vi "HK Channel Setup and Test.vi"() -> ()   [LabVIEW 2019]
uses:
  HK Table/HK Current Value Table Settings.ctl
  HK Item/HK Channel Units and Setup.ctl
  HK Item/HK Channel enum Data Type.ctl
  HK Item/HK Channel Settings Physical.ctl
  HK Item/HK Channel Settings Scaling.ctl
  HK Item/HK Channel enum Scaling Type.ctl
  HK Item/HK Channel Settings Limits.ctl
  HK Alarms/HK Channel Settings Alarms.ctl
  HK Alarms/HK Alarm enum Action.ctl
  HK Table/HK Table.lvclass
  HK Item/HK Item.lvclass
  HK Table/HK Table.lvclass/HK Table.ctl
  HK Item/HK Item.lvclass/HK Item.ctl
  HK Alarms/HK Alarms.lvclass/HK Alarms.ctl
  HK Item/HK Channel Read Name.vi
  HK Table/HK Channel Write Channel Configuration File.vi
  HK Alarms/HK Alarms.lvclass
panel:
  in  "Channels":i32(listbox)
  in  "Tab Control":T1(tab)
  in  "Channel List":i32(listbox)
  in  "CVT Settings":T2 {"Max Age" format="%<%H:%M:%S>t"}
  in  "HK File":string
  in  "Save Button":bool
  in  "Update Ch":bool
  in  "Channel Name":string
  in  "Channel Setup":T3
  in  "Add Channel":bool
  in  "Update Phy":bool
  in  "Physical":T5
  in  "Scaling":T6
  in  "Update Alarms":bool
  in  "Limits":T8
  in  "Alarms":T9[](array[typedef])
  in  "Delete Channel":bool
  in  "Close":bool
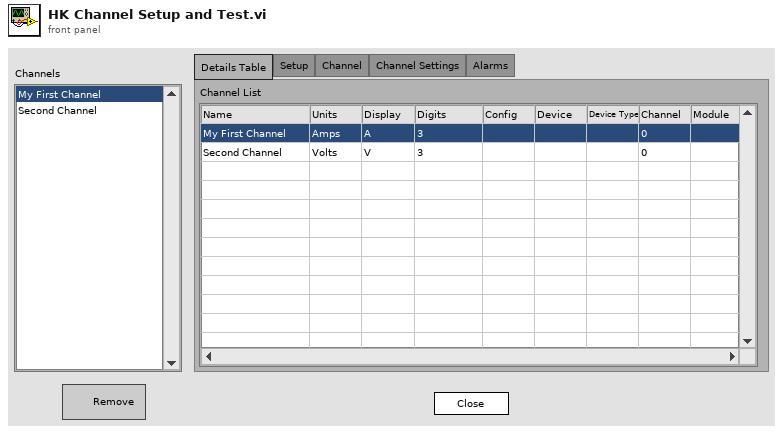
[diagram p1: front panel]
types:
  T1 = enum32{"Details Table", "Setup", "Channel", "Channel Settings", "Alarms"}
  T2 = typedef "HK Table.lvclass/HK Current Value Table Settings.ctl" = cluster{"Running Avg Elements":i32, "Max Age":dbl}
  T3 = typedef "HK Item.lvclass/HK Channel Units and Setup.ctl" = cluster{"Unit Type":string, "Units":string, "Configuration":string, "Digits":i32, "Data Type":T4}
  T4 = typedef "HK Item.lvclass/HK Channel enum Data Type.ctl" = enum16{"Floating Point", "Integer", "Enum", "String", "Waveform", "File"}
  T5 = typedef "HK Item.lvclass/HK Channel Settings Physical.ctl" = cluster{"Type":string, "Device":string, "Module":string, "Channel":i32}
  T6 = typedef "HK Item.lvclass/HK Channel Settings Scaling.ctl" = cluster{"Scaling Type":T7, "Parameters":dbl[]}
  T7 = typedef "HK Item.lvclass/HK Channel enum Scaling Type.ctl" = enum16{"None", "Polynomial"}
  T8 = typedef "HK Item.lvclass/HK Channel Settings Limits.ctl" = cluster{"Low Red":dbl, "Low Yellow":dbl, "Hi Yellow":dbl, "Hi Red":dbl}
  T9 = typedef "HK Item.lvclass/HK Channel Settings Alarms.ctl" = cluster{"Enabled":bool, "Deadband":i32, "Action":T10}
  T10 = typedef "HK Item.lvclass/HK Alarm enum Action.ctl" = enum16{"Light", "Message", "Safe"}
  T11 = cluster{"state":refnum<user-event>, "HK Channels":refnum<class "HK Table.lvclass">, "Channel Ref":refnum<class "HK Item.lvclass">}
  T12 = typedef "HK cluster Create Defaults.ctl" = cluster{"HK File":string, "CVT Settings":T2}
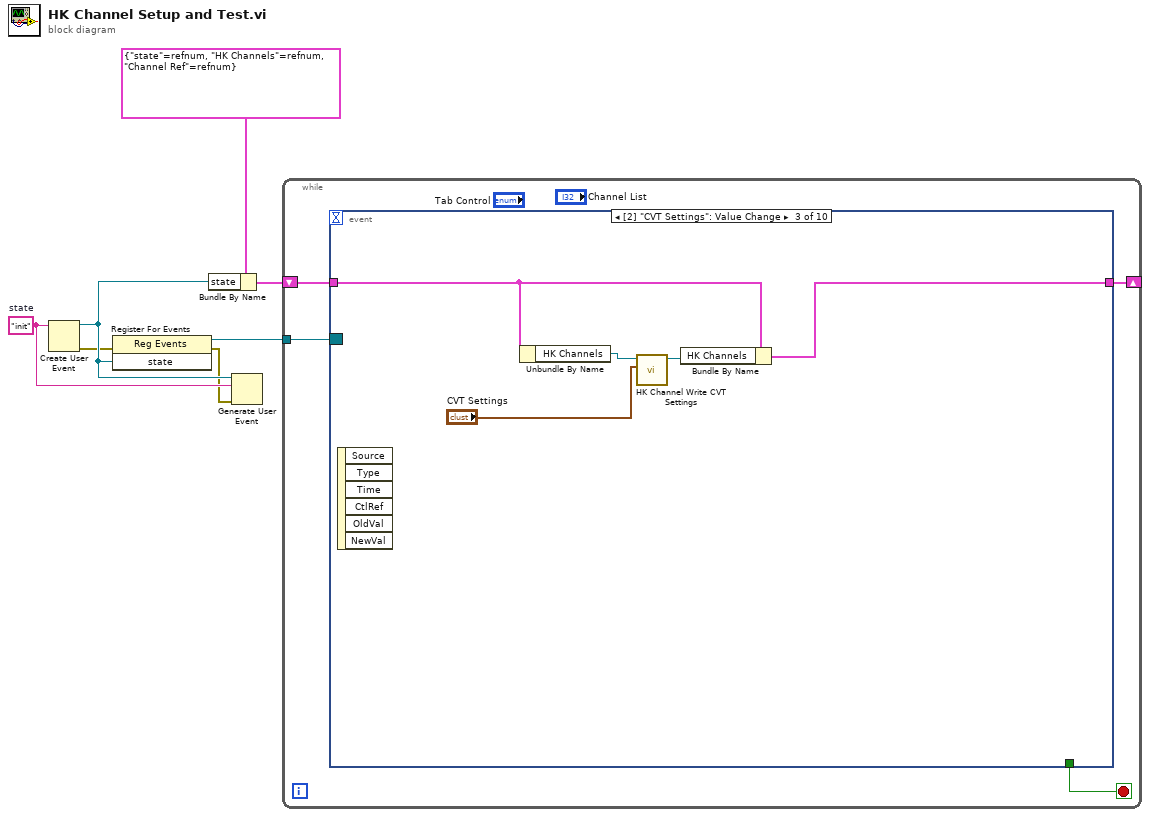
[diagram p0: block diagram]
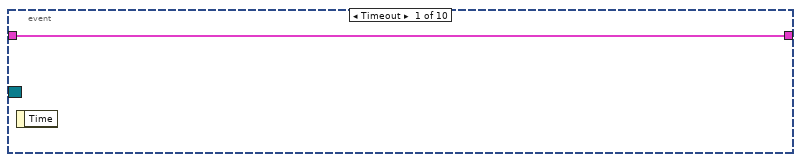
[diagram p2: hidden frame]
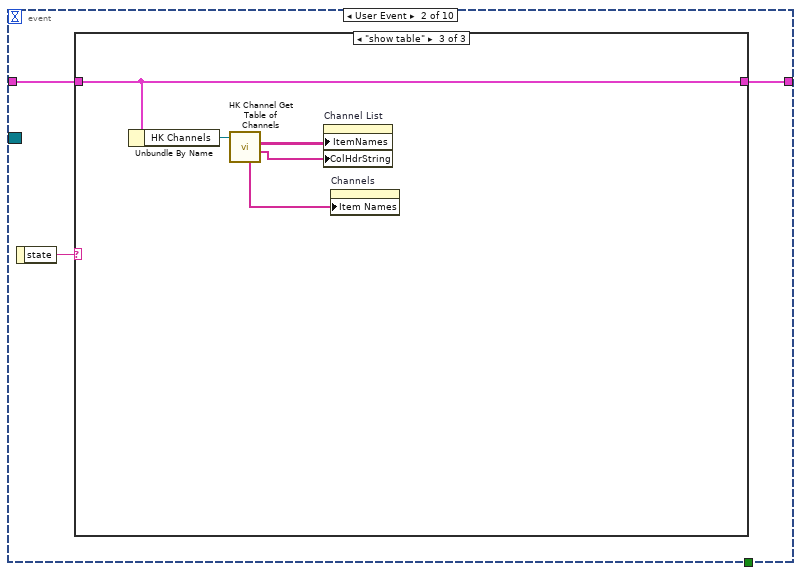
[diagram p3: hidden frame]
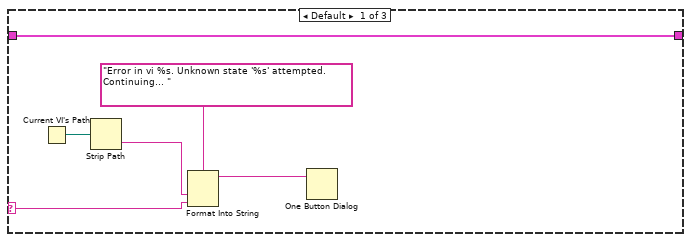
[diagram p4: hidden frame]
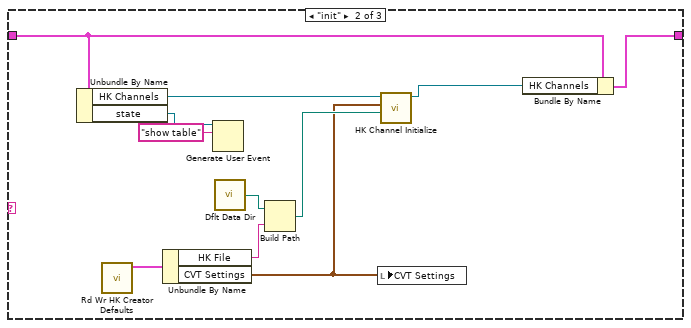
[diagram p5: hidden frame]
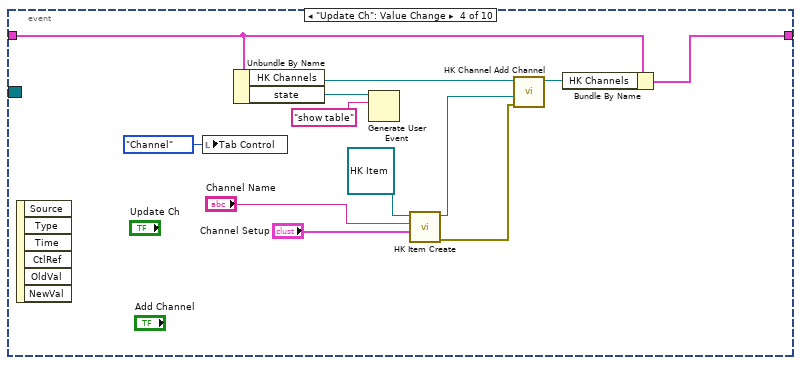
[diagram p6: hidden frame]
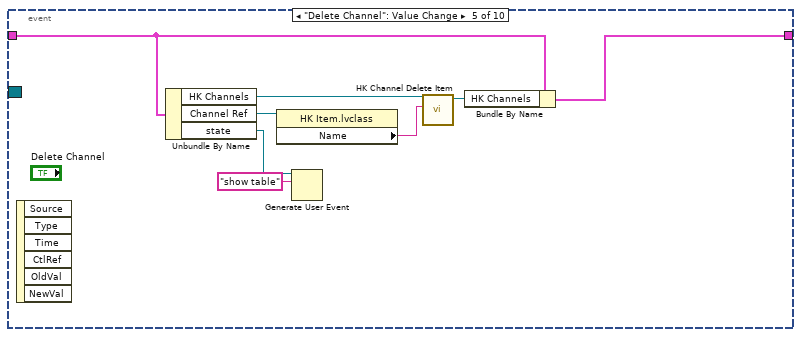
[diagram p7: hidden frame]
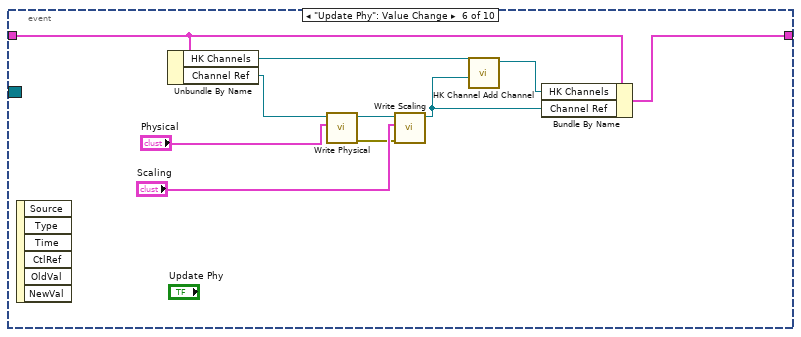
[diagram p8: hidden frame]
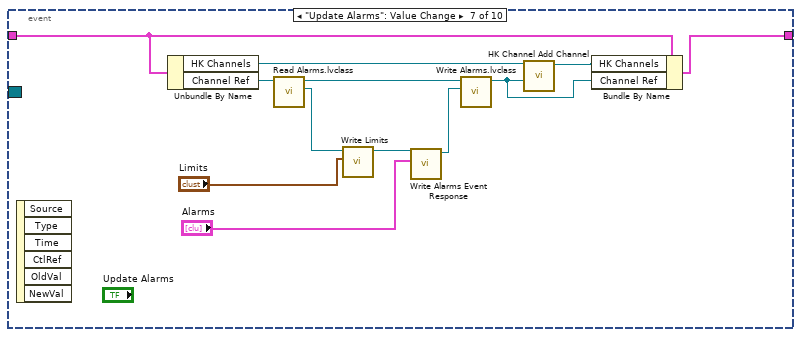
[diagram p9: hidden frame]
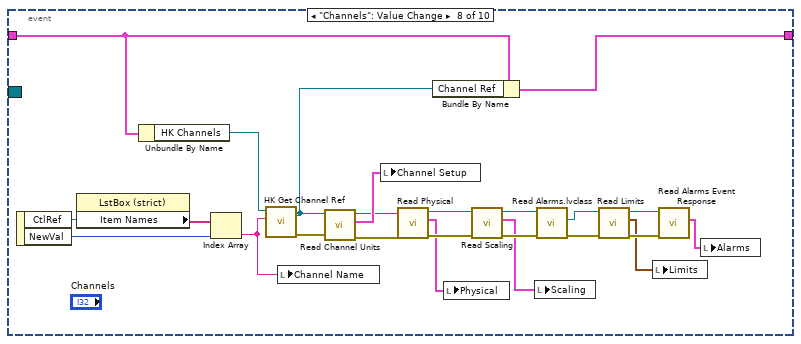
[diagram p10: hidden frame]
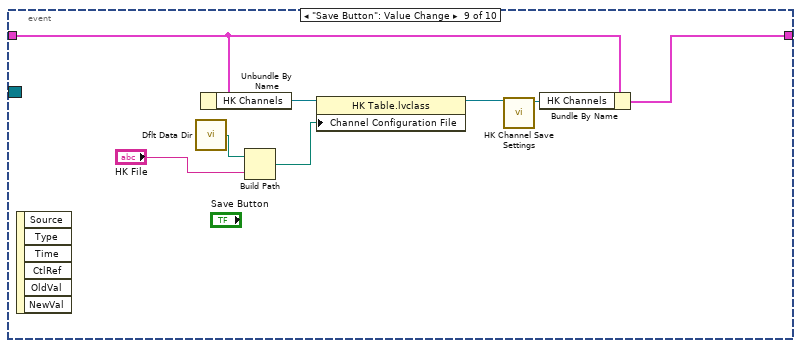
[diagram p11: hidden frame]
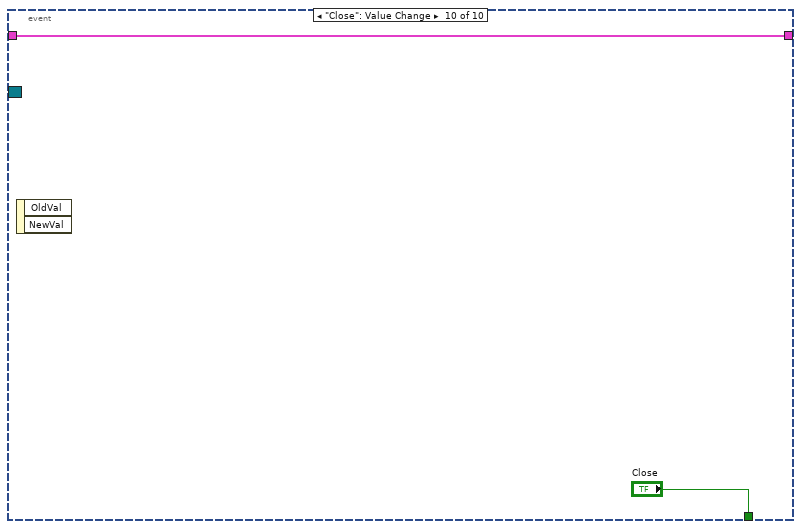
[diagram p12: hidden frame]
diagram:
  w3 = "init"  # state
  n1 = Create User Event(user event datatype=w3) -> (user event=w5:refnum<user-event>, error out=w1:errorcluster)  [unwired: 1 in]
  n2 = register-events(error in=w1, w5) -> (reference out=w4:refnum<event-registration>, error out=w2:errorcluster)  [unwired: 1 in]
  n3 = Bundle By Name(cluster=T11 {"state"=refnum, "HK Channels"=refnum, "Channel Ref"=refnum}, "state"=w5) -> (w6:T11)
  n4 = Generate User Event(user event=w5, event data cluster=w3, error in=w2) -> ()  [unwired: 1 in, 2 out]
  n5 = while {
    tunnel: w4 -> [w11]
    shift-right: [w9] -> _
    shift-left: w6 -> [w10]
    stop <- w8 stop-if-true
    n6 = event shown="[2] \"CVT Settings\": Value Change" {
      selector: w11 -> [_ _ _ _ _ _ _ _ _ _]
      dyn-events: _ -> [_ _ _ _ _ _ _ _ _ _]
      timeout: _ -> [_ _ _ _ _ _ _ _ _ _]
      tunnel: w10 -> [w12 w14 w38 w45 w57 w66 w74 w91 w109 w118]
      tunnel: [w12 w13 w39 w46 w58 w67 w73 w92 w110 w118] -> w9
      tunnel: [_ _ _ _ _ _ _ _ _ "Close"] -> w8
      event Timeout {
        n7 = event-data() -> ()  [unwired: 1 in, 1 out]
      }
      event User Event {
        n8 = event-data() -> ("state"=w15:string)  [unwired: 1 in]
        n9 = case shown="\"show table\"" w15 {
          selector: w15 -> [w20 _ _]
          tunnel: w14 -> [w16 w29 w37]
          tunnel: [w16 w30 w37] -> w13
          frame Default {
            n10 = Current VI's Path() -> (path=w19:path)
            n11 = Strip Path(path=w19) -> (name=w18:string)  [unwired: 1 out]
            n12 = Format Into String(format string="Error in vi %s. Unknown state '%s' attempted. Continuing... ", w18, w20) -> (resulting string=w17:string)  [unwired: 2 in, 1 out]
            n13 = One Button Dialog(message=w17) -> ()  [unwired: 1 in, 1 out]
          }
          frame "init" {
            n14 = Unbundle By Name(w29) -> ("HK Channels"=w32:refnum<class "HK Table.lvclass">, "state"=w28:refnum<user-event>)
            n15 = call "Rd Wr HK Creator Defaults.vi"() -> ("HK Creator Defaults"=w26:T12)  [unwired: 10 in, 1 out]
            n16 = Unbundle By Name(w26) -> ("HK File"=w24:string, "CVT Settings"=w22:T2)
            n17 = Generate User Event(user event=w28, event data cluster="show table" ("event data")) -> ()  [unwired: 2 in, 2 out]
            n18 = call <vilib>:"Dflt Data Dir.vi"() -> ("App:Default Data Directory"=w25:path)
            n19 = Build Path(base path=w25, name or relative path=w24) -> (appended path=w23:path)
            n20 = local write "CVT Settings"(w22) -> ()
            n21 = call-dynamic "HK Channel Initialize.vi"("Channel Configuration File"=w23, "CVT Settings"=w22, "HK Channel in"=w32) -> ("HK Channel out"=w31:refnum<class "HK Table.lvclass">)  [unwired: 7 in, 1 out]
            n22 = Bundle By Name(cluster=w29, "HK Channels"=w31) -> (w30:T11)
          }
          frame "show table" {
            n23 = Unbundle By Name(w37) -> ("HK Channels"=w36:refnum<class "HK Table.lvclass">)
            n24 = call-dynamic "HK Channel Get Table of Channels.vi"("HK Channel in"=w36) -> ("Header"=w33:string[], "Table"=w35:string[][], "Ch Names"=w34:string[])  [unwired: 6 in, 2 out]
            n25 = property on="Channel List" class="MCListbox (strict)"("ItemNames"=w35, "ColHdrString"=w33) -> ()  [unwired: 2 in, 2 out]
            n26 = property on="Channels" class="LstBox (strict)"("Item Names"=w34) -> ()  [unwired: 2 in, 2 out]
          }
        }
      }
      event Value Change {
        n27 = event-data() -> ()  [unwired: 1 in, 6 out]
        n28 = Unbundle By Name(w38) -> ("HK Channels"=w42:refnum<class "HK Table.lvclass">)
        n29 = call "HK Channel Write CVT Settings.vi"("CVT Settings"="CVT Settings", "HK Channel in"=w42) -> ("HK Channel out"=w40:refnum<class "HK Table.lvclass">)  [unwired: 8 in, 1 out]
        n30 = Bundle By Name(cluster=w38, "HK Channels"=w40) -> (w39:T11)
      }
      event "Update Ch": Value Change {
        n31 = event-data() -> ()  [unwired: 1 in, 6 out]
        n32 = local write "Tab Control"(enum32{"Details Table", "Setup", "Channel"}."Channel" ("Tab Control")) -> ()
        n33 = Unbundle By Name(w45) -> ("HK Channels"=w51:refnum<class "HK Table.lvclass">, "state"=w44:refnum<user-event>)
        n34 = Generate User Event(user event=w44, event data cluster="show table" ("event data")) -> ()  [unwired: 2 in, 2 out]
        n35 = call-dynamic "HK Item Create.vi"("Channel Setup"="Channel Setup", "Name"="Channel Name", "HK Item in"=refnum<class "HK Item.lvclass"> refnum) -> ("error out"=w48:errorcluster, "HK Item out"=w50:refnum<class "HK Item.lvclass">)  [unwired: 7 in]
        n36 = call-dynamic "HK Channel Add Channel.vi"("error in (no error)"=w48, "HK Item.lvclass"=w50, "HK Channel in"=w51) -> ("HK Channel out"=w47:refnum<class "HK Table.lvclass">)  [unwired: 7 in, 1 out]
        n37 = Bundle By Name(cluster=w45, "HK Channels"=w47) -> (w46:T11)
      }
      event "Delete Channel": Value Change {
        n38 = event-data() -> ()  [unwired: 1 in, 6 out]
        n39 = Unbundle By Name(w57) -> ("HK Channels"=w61:refnum<class "HK Table.lvclass">, "Channel Ref"=w62:refnum<class "HK Item.lvclass">, "state"=w56:refnum<user-event>)
        n40 = property class="HK Item.lvclass"(reference=w62) -> ("Name"=w60:string)  [unwired: 1 in, 2 out]
        n41 = Generate User Event(user event=w56, event data cluster="show table" ("event data")) -> ()  [unwired: 2 in, 2 out]
        n42 = call-dynamic "HK Channel Delete Item.vi"("Channel Name"=w60, "HK Channel in"=w61) -> ("HK Channel out"=w59:refnum<class "HK Table.lvclass">)  [unwired: 6 in, 3 out]
        n43 = Bundle By Name(cluster=w57, "HK Channels"=w59) -> (w58:T11)
      }
      event "Update Phy": Value Change {
        n44 = event-data() -> ()  [unwired: 1 in, 6 out]
        n45 = Unbundle By Name(w66) -> ("HK Channels"=w65:refnum<class "HK Table.lvclass">, "Channel Ref"=w72:refnum<class "HK Item.lvclass">)
        n46 = call "Write Physical.vi"("Physical"="Physical", "HK Item in"=w72) -> ("error out"=w68:errorcluster, "HK Item out"=w70:refnum<class "HK Item.lvclass">)  [unwired: 8 in]
        n47 = call "Write Scaling.vi"("error in (no error)"=w68, "Scaling"="Scaling", "HK Item in"=w70) -> ("HK Item out"=w64:refnum<class "HK Item.lvclass">)  [unwired: 7 in, 1 out]
        n48 = call-dynamic "HK Channel Add Channel.vi"("HK Item.lvclass"=w64, "HK Channel in"=w65) -> ("HK Channel out"=w63:refnum<class "HK Table.lvclass">)  [unwired: 8 in, 1 out]
        n49 = Bundle By Name(cluster=w66, "HK Channels"=w63, "Channel Ref"=w64) -> (w67:T11)
      }
      event "Update Alarms": Value Change {
        n50 = event-data() -> ()  [unwired: 1 in, 6 out]
        n51 = Unbundle By Name(w74) -> ("HK Channels"=w84:refnum<class "HK Table.lvclass">, "Channel Ref"=w79:refnum<class "HK Item.lvclass">)
        n52 = call "Read Alarms.lvclass.vi"("HK Item in"=w79) -> ("Alarms.lvclass"=w78:refnum<class "HK Alarms.lvclass">, "HK Item out"=w76:refnum<class "HK Item.lvclass">)  [unwired: 8 in, 1 out]
        n53 = call "Write Limits.vi"("Limits"="Limits", "Alarms in"=w78) -> ("Alarms out"=w80:refnum<class "HK Alarms.lvclass">)  [unwired: 8 in, 1 out]
        n54 = call "Write Alarms Event Response.vi"("Alarms"="Alarms", "Alarms in"=w80) -> ("Alarms out"=w77:refnum<class "HK Alarms.lvclass">)  [unwired: 8 in, 1 out]
        n55 = call "Write Alarms.lvclass.vi"("Alarms.lvclass"=w77, "HK Item in"=w76) -> ("HK Item out"=w75:refnum<class "HK Item.lvclass">)  [unwired: 8 in, 1 out]
        n56 = call-dynamic "HK Channel Add Channel.vi"("HK Item.lvclass"=w75, "HK Channel in"=w84) -> ("HK Channel out"=w83:refnum<class "HK Table.lvclass">)  [unwired: 8 in, 1 out]
        n57 = Bundle By Name(cluster=w74, "HK Channels"=w83, "Channel Ref"=w75) -> (w73:T11)
      }
      event "Channels": Value Change {
        n58 = event-data() -> ("CtlRef"=w108:refnum<vi>, "NewVal"=w106:i32)  [unwired: 1 in]
        n59 = property class="LstBox (strict)"(reference=w108) -> ("Item Names"=w107:string[])  [unwired: 1 in, 2 out]
        n60 = Unbundle By Name(w91) -> ("HK Channels"=w105:refnum<class "HK Table.lvclass">)
        n61 = Index Array(array=w107, index=w106) -> (element=w90:string)
        n62 = call-dynamic "HK Get Channel Ref.vi"("Channel Name"=w90, "HK Channel in"=w105) -> ("error out"=w87:errorcluster, "Channel Ref"=w89:refnum<class "HK Item.lvclass">)  [unwired: 7 in, 1 out]
        n63 = local write "Channel Name"(w90) -> ()
        n64 = call "Read Channel Units.vi"("error in (no error)"=w87, "HK Item in"=w89) -> ("error out"=w85:errorcluster, "Channel Setup"=w88:T3, "HK Item out"=w86:refnum<class "HK Item.lvclass">)  [unwired: 7 in]
        n65 = local write "Channel Setup"(w88) -> ()
        n66 = call "Read Physical.vi"("error in (no error)"=w85, "HK Item in"=w86) -> ("error out"=w103:errorcluster, "Physical"=w96:T5, "HK Item out"=w104:refnum<class "HK Item.lvclass">)  [unwired: 7 in]
        n67 = Bundle By Name(cluster=w91, "Channel Ref"=w89) -> (w92:T11)
        n68 = local write "Physical"(w96) -> ()
        n69 = call "Read Scaling.vi"("error in (no error)"=w103, "HK Item in"=w104) -> ("error out"=w101:errorcluster, "Scaling"=w95:T6, "HK Item out"=w102:refnum<class "HK Item.lvclass">)  [unwired: 7 in]
        n70 = local write "Scaling"(w95) -> ()
        n71 = call "Read Alarms.lvclass.vi"("error in (no error)"=w101, "HK Item in"=w102) -> ("error out"=w99:errorcluster, "Alarms.lvclass"=w100:refnum<class "HK Alarms.lvclass">)  [unwired: 7 in, 1 out]
        n72 = call "Read Limits.vi"("error in (no error)"=w99, "Alarms in"=w100) -> ("error out"=w97:errorcluster, "Limits"=w94:T8, "Alarms out"=w98:refnum<class "HK Alarms.lvclass">)  [unwired: 7 in]
        n73 = local write "Limits"(w94) -> ()
        n74 = call "Read Alarms Event Response.vi"("error in (no error)"=w97, "Alarms in"=w98) -> ("Alarms"=w93:T9[])  [unwired: 7 in, 2 out]
        n75 = local write "Alarms"(w93) -> ()
      }
      event "Save Button": Value Change {
        n76 = event-data() -> ()  [unwired: 1 in, 6 out]
        n77 = call <vilib>:"Dflt Data Dir.vi"() -> ("App:Default Data Directory"=w115:path)
        n78 = Unbundle By Name(w109) -> ("HK Channels"=w116:refnum<class "HK Table.lvclass">)
        n79 = Build Path(base path=w115, name or relative path="HK File") -> (appended path=w112:path)
        n80 = property class="HK Table.lvclass"(reference=w116, "Channel Configuration File"=w112) -> (reference out=w113:refnum<class "HK Table.lvclass">)  [unwired: 1 in, 1 out]
        n81 = call-dynamic "HK Channel Save Settings.vi"("HK Channel in"=w113) -> ("HK Channel out"=w111:refnum<class "HK Table.lvclass">)  [unwired: 8 in, 2 out]
        n82 = Bundle By Name(cluster=w109, "HK Channels"=w111) -> (w110:T11)
      }
      event "Close": Value Change {
        n83 = event-data() -> ()  [unwired: 1 in, 2 out]
      }
    }
  }
